vi "call_MB_TCP.vi"(5 "Status Reference":T2, 6 "N":i32, 7 "Data Reference":T1, 8 "error in":errorcluster, 9 "timeouts":T3={"conn_timeout"=1000, "reconn_timeout"=3000, "N attempt max"=3, "t_reset_TTL"=120000, "write_timeout"=10, "read_timeout"=500, "period"=100} {"t_reset_TTL" min=10 max=240000 step=1; "period" min=10 max=100000 step=1; "read_timeout" min=10 max=60000 step=1; "write_timeout" min=1 max=60000 step=1; "N attempt max" min=1 max=5 step=1; "reconn_timeout" min=10 max=240000 step=1; "conn_timeout" min=10 max=240000}, 10 "Module Name":string="MB_TCP_ZERO_p.vi") -> (0 "error out":errorcluster, 3 "vi reference":refnum<vi>)   [LabVIEW 2019, in "MB_TCP1.lvlib"]
uses:
  MB_TCP1.lvlib
  ICPCON Status/Ctl/ICPCON Status.ctl
  ICPCON Registers/Ctl/ICPCON Data.ctl
  ICPCON Status/ICPCON Status.lvlib
  ICPCON Registers/ICPCON Registers.lvlib
panel:
  # "VI Name:\nPurpose: Dynamically calls *.vi"
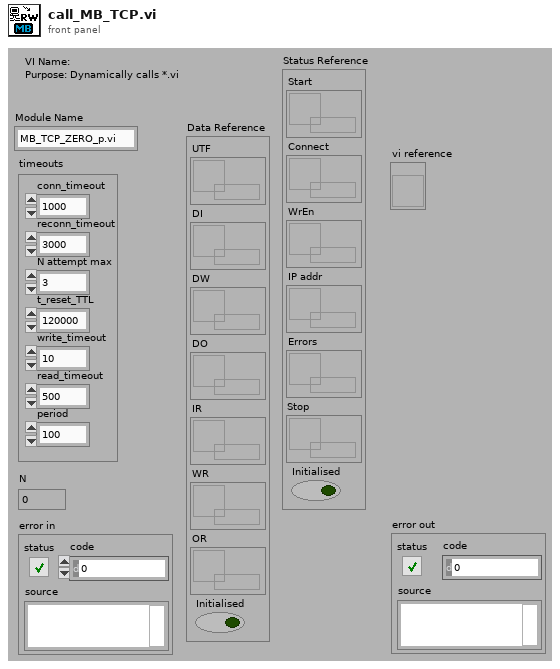
[diagram p1: front panel]
types:
  T1 = typedef "ICPCON Registers.lvlib/ICPCON Data.ctl" = cluster{"UTF":refnum<data-value>, "DI":refnum<data-value>, "DW":refnum<data-value>, "DO":refnum<data-value>, "IR":refnum<data-value>, "WR":refnum<data-value>, "OR":refnum<data-value>, "Initialised":bool}
  T2 = typedef "ICPCON Status.lvlib/ICPCON Status.ctl" = cluster{"Start":refnum<data-value>, "Connect":refnum<data-value>, "WrEn":refnum<data-value>, "IP addr":refnum<data-value>, "Errors":refnum<data-value>, "Stop":refnum<data-value>, "Initialised":bool}
  T3 = cluster{"conn_timeout":i32, "reconn_timeout":i32, "N attempt max":i32, "t_reset_TTL":i32, "write_timeout":i32, "read_timeout":i32, "period":i32}
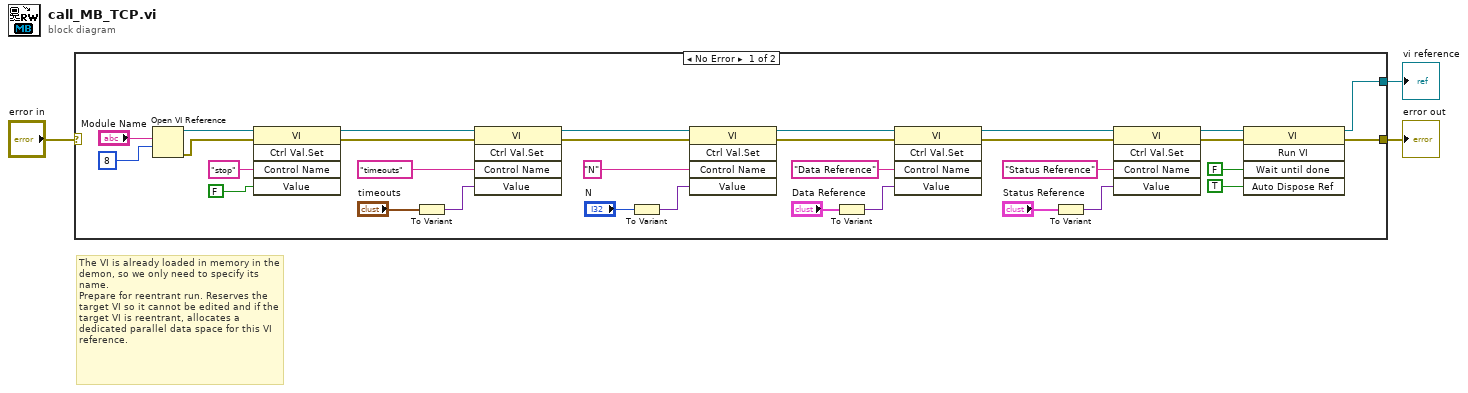
[diagram p0: block diagram]
diagram:
  # "The VI is already loaded in memory in the demon, so we only need to specify its name.\nPrepare for reentrant run. Reserves the target VI so it cannot be edited and if the target VI is reentrant, allocates a dedicated parallel data space for this VI reference."
  n1 = case shown="No Error" "error in" {
    selector: "error in" -> [_ w36]
    tunnel: [w24 w36] -> w3
    tunnel: [w10 _] -> w2
    frame No Error {
      n2 = Open VI Reference(vi path="Module Name", options=8) -> (vi reference=w7:refnum<vi>, error out=w5:errorcluster)  [unwired: 4 in]
      n3 = invoke class="VI" method="Ctrl Val.Set"(reference=w7, error in=w5, "Control Name"="stop", "Value"=FALSE) -> (reference out=w6:refnum<vi>, error out=w4:errorcluster)  [unwired: 1 in, 3 out]
      n4 = To Variant(anything="timeouts") -> (Variant=w33:variant)
      n5 = invoke class="VI" method="Ctrl Val.Set"(reference=w6, error in=w4, "Control Name"="timeouts", "Value"=w33) -> (reference out=w23:refnum<vi>, error out=w28:errorcluster)  [unwired: 1 in, 3 out]
      n6 = To Variant(anything="N") -> (Variant=w29:variant)
      n7 = invoke class="VI" method="Ctrl Val.Set"(reference=w23, error in=w28, "Control Name"="N", "Value"=w29) -> (reference out=w17:refnum<vi>, error out=w16:errorcluster)  [unwired: 1 in, 3 out]
      n8 = To Variant(anything="Data Reference") -> (Variant=w22:variant)
      n9 = invoke class="VI" method="Ctrl Val.Set"(reference=w17, error in=w16, "Control Name"="Data Reference", "Value"=w22) -> (reference out=w14:refnum<vi>, error out=w12:errorcluster)  [unwired: 1 in, 3 out]
      n10 = To Variant(anything="Status Reference") -> (Variant=w19:variant)
      n11 = invoke class="VI" method="Ctrl Val.Set"(reference=w14, error in=w12, "Control Name"="Status Reference", "Value"=w19) -> (reference out=w13:refnum<vi>, error out=w11:errorcluster)  [unwired: 1 in, 3 out]
      n12 = invoke class="VI" method="Run VI"(reference=w13, error in=w11, "Wait until done"=FALSE, "Auto Dispose Ref"=TRUE) -> (reference out=w10:refnum<vi>, error out=w24:errorcluster)  [unwired: 1 in, 3 out]
    }
    frame Error {
    }
  }
  "error out" <- w3
  "vi reference" <- w2
